vi "Debug - IP and Port Placeholder--Const.vi"() -> (3 "Debug Placeholder":string)   [LabVIEW 2017, in "Communications Library.lvlib"]
uses:
  Communications Library.lvlib
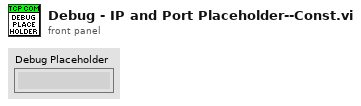
[diagram p1: front panel]
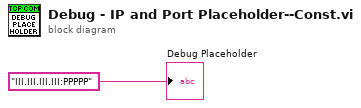
[diagram p0: block diagram]
diagram:
  "Debug Placeholder" <- "III.III.III.III:PPPPP" ("data in")
